vi "auto match.vi"() -> ()   [LabVIEW 2014]
panel:
  out "current number":dbl format="%#.0f"
  out "# of iterations":i32
  in  "number to match":dbl=50.0 min=0.0 max=1000.0 step=1.0 format="%#.0f"
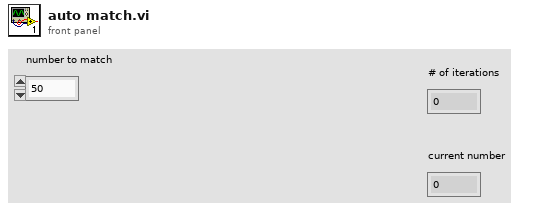
[diagram p1: front panel]
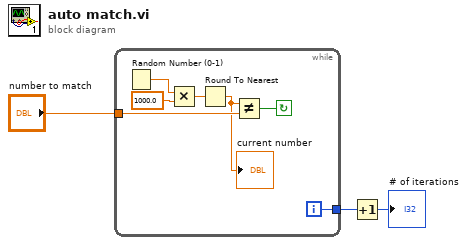
[diagram p0: block diagram]
diagram:
  n1 = while {
    tunnel: "number to match" -> [w7]
    tunnel: [w4] -> w1
    i -> [w4]
    stop <- w5 continue-if-true
    n2 = Random Number (0-1)() -> (number: 0 to 1=w10:dbl)
    n3 = Multiply(x=w10, y=1000.0) -> (x*y=w8:dbl)
    n4 = Round To Nearest(number=w8) -> (nearest integer value=w6:dbl)
    "current number" <- w6
    n5 = Not Equal?(x=w6, y=w7) -> (x != y?=w5:bool)
  }
  n6 = Increment(x=w1) -> (x+1=→"# of iterations":i32)
